vi "Simulate Keyboard.vi"(8 "error in (no error)":errorcluster, 10 "Virtual Key":u8(ring)=65, 11 "Action":enum16{"Key Down", "Key Up"}(ring)) -> (0 "error out":errorcluster)   [LabVIEW 2017]
doc: "This VI allows you to simulate a keyboard action. To perform a press you would need to execute this VI twice, once with key down, then with key up."
uses:
  User32.dll
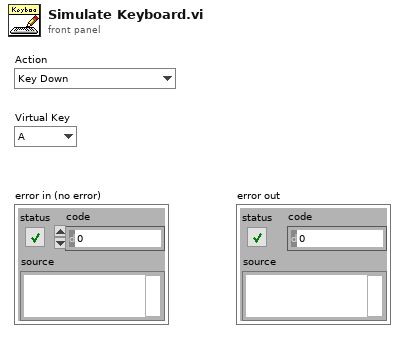
[diagram p1: front panel]
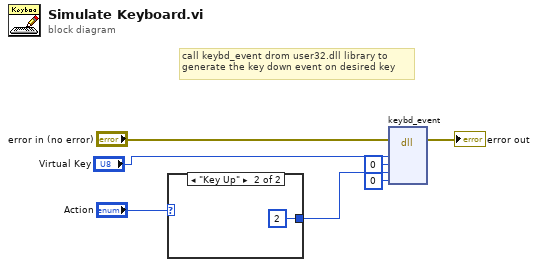
[diagram p0: block diagram]
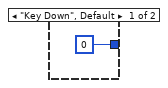
[diagram p2: hidden frame]
diagram:
  # "call keybd_event drom user32.dll library to \ngenerate the key down event on desired key"
  n1 = case shown="\"Key Up\"" "Action" {
    tunnel: [u32 0 u32 2] -> w1
    frame "Key Down", Default {
    }
    frame "Key Up" {
    }
  }
  n2 = dll-call lib="user32.dll" fn="keybd_event"(error in="error in (no error)", "bVk"="Virtual Key", "bScan"=u8 0, "dwFlags"=w1, "dwExtraInfo"=u32 0) -> (error out=→"error out":errorcluster)  [unwired: 7 in, 1 out]
